vi "Get error (sp-pv).vi"(2 "options":T1={"sp low"=0.0, "sp high"=100.0, "out low"=-100.0, "out high"=100.0, "hold (F)"=FALSE, "auto (T)"=TRUE, "pro. band (F)"=FALSE, "reverse acting (T)"=TRUE, "beta"=1.0, "linearity"=1.0, "dt (s)"=-1.0} {"dt (s)" format="%.2f"; "linearity" min=0.0 max=1.0 format="%.2f"; "sp low" format="%.2f"; "sp high" format="%.2f"; "out low" format="%.2f"; "out high" format="%.2f"; "beta" min=0.0 max=1.0 format="%.2f"}, 3 "process variable":dbl format="%.2f", 4 "setpoint":dbl format="%.2f") -> (0 "error":dbl format="%.2f", 1 "error (with beta)":dbl format="%.2f")   [LabVIEW 2017, in "NI_PID__prctrl compat.lvlib"]
doc: "This function calculates the error between the process variable and setpoint value. The error (with beta) output is used for the proportional action and the error output is used for the integral action."
uses:
  <vilib>/addons/control/pid/NI_PID__prctrl compat.lvlib
panel:
  # "SP & PV range:"
  # "Output range:"
  # "-1: default,using\nsystem clock"
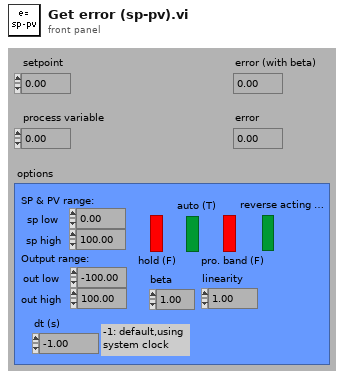
[diagram p1: front panel]
types:
  T1 = cluster{"sp low":dbl, "sp high":dbl, "out low":dbl, "out high":dbl, "hold (F)":bool, "auto (T)":bool, "pro. band (F)":bool, "reverse acting (T)":bool, "beta":dbl, "linearity":dbl, "dt (s)":dbl}
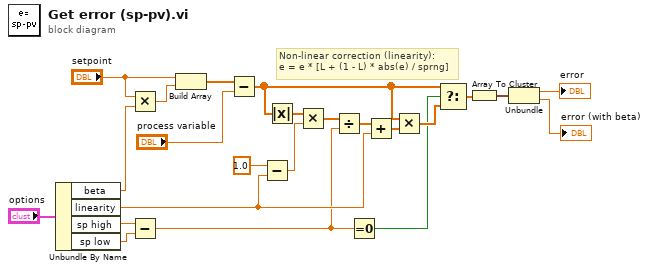
[diagram p0: block diagram]
diagram:
  # "Non-linear correction (linearity):\ne = e * [L + (1 - L) * abs(e) / sprng]"
  n1 = Unbundle By Name("options") -> ("beta"=w19:dbl, "linearity"=w10:dbl, "sp high"=w22:dbl, "sp low"=w21:dbl)
  n2 = Multiply(x="setpoint", y=w19) -> (x*y=w18:dbl)
  n3 = Subtract(x=w22, y=w21) -> (x-y=w5:dbl)
  n4 = Build Array("setpoint", w18) -> (w15:dbl[])
  n5 = Subtract(x=w15, y="process variable") -> (x-y=w3:dbl[])
  n6 = Subtract(x=1.0, y=w10) -> (x-y=w13:dbl)
  n7 = Absolute Value(x=w3) -> (abs(x)=w14:dbl[])
  n8 = Multiply(x=w14, y=w13) -> (x*y=w12:dbl[])
  n9 = Divide(x=w12, y=w5) -> (x/y=w11:dbl[])
  n10 = Equal To 0?(x=w5) -> (x = 0?=w1:bool)
  n11 = Add(x=w11, y=w10) -> (x+y=w9:dbl[])
  n12 = Multiply(x=w3, y=w9) -> (x*y=w2:dbl[])
  n13 = Select(t=w3, s=w1, f=w2) -> (s? t:f=w4:dbl[])
  n14 = Array To Cluster(array=w4) -> (cluster=w8:cluster{"[0]":dbl, "[1]":dbl})
  n15 = Unbundle(w8) -> ("[0]"=→"error":dbl, "[1]"=→"error (with beta)":dbl)
